vi "Start.vi"(8 "error in (no error)":errorcluster, 10 "Message in":refnum<class "StartMessage.lvclass">, 11 "ExampleClassA in":refnum<class "ExampleClassA.lvclass">) -> (0 "error out":errorcluster, 3 "ExampleClassA out":refnum<class "ExampleClassA.lvclass">)   [LabVIEW 2012, in "ExampleClassA.lvclass"]
doc: "Starts the data production and streaming to observers."
uses:
  ExampleClassA.lvclass
  <vilib>/Distrio/Murmex/StartMessage/StartMessage.lvclass
  <vilib>/Distrio/Murmex/Murmex/Murmex.lvclass
  <vilib>/Distrio/Murmex/ProceedMessage/ProceedMessage.lvclass
  ExampleClassA.lvclass/ExampleClassA.ctl
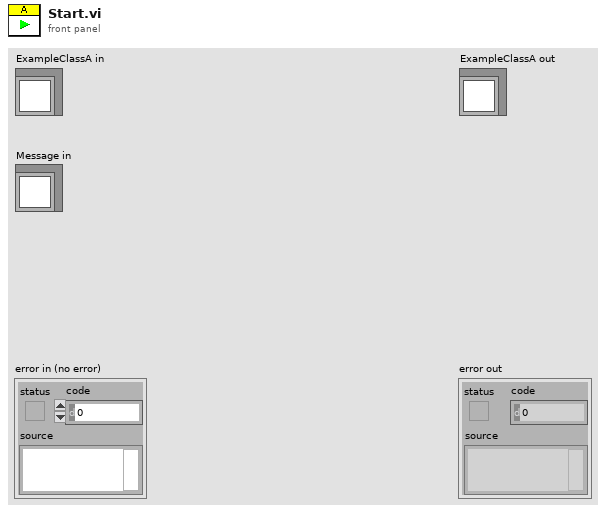
[diagram p1: front panel]
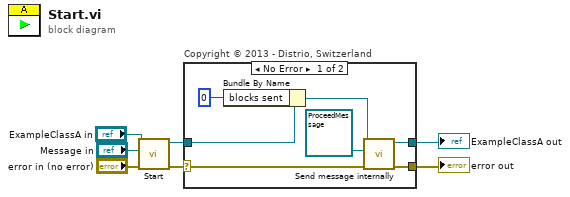
[diagram p0: block diagram]
diagram:
  n1 = call-parent "Start.vi"("error in (no error)"="error in (no error)", "Message in"="Message in", "Murmex in"="ExampleClassA in") -> ("error out"=w1:errorcluster, "Murmex out"=w5:refnum<class "ExampleClassA.lvclass">)  [unwired: 7 in]
  n2 = case "Copyright © 2013 - Distrio, Switzerland" shown="No Error" w1 {
    selector: w1 -> [w8 w15]
    tunnel: w5 -> [w14 w16]
    tunnel: [w13 w16] -> w4
    tunnel: [w10 w15] -> w3
    frame No Error {
      n3 = Bundle By Name(cluster=w14, "blocks sent"=0 ("internal state.samples read")) -> (w11:refnum<class "ExampleClassA.lvclass">)
      n4 = call <vilib>:"Send message internally.vi"("error in (no error)"=w8, "Message"=refnum<class "ProceedMessage.lvclass"> refnum ("Distrio Murmex 1.5:ProceedMessage"), "Murmex in"=w11) -> ("error out"=w10:errorcluster, "Murmex out"=w13:refnum<class "ExampleClassA.lvclass">)  [unwired: 7 in]
    }
    frame Error {
    }
  }
  "error out" <- w3
  "ExampleClassA out" <- w4
